vi "ParseData (SubVI).vi"(11 "read buffer":string) -> (3 "Array":bool[][](array[boolean]))   [LabVIEW 2021]
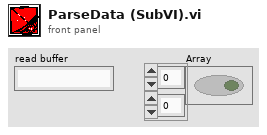
[diagram p1: front panel]
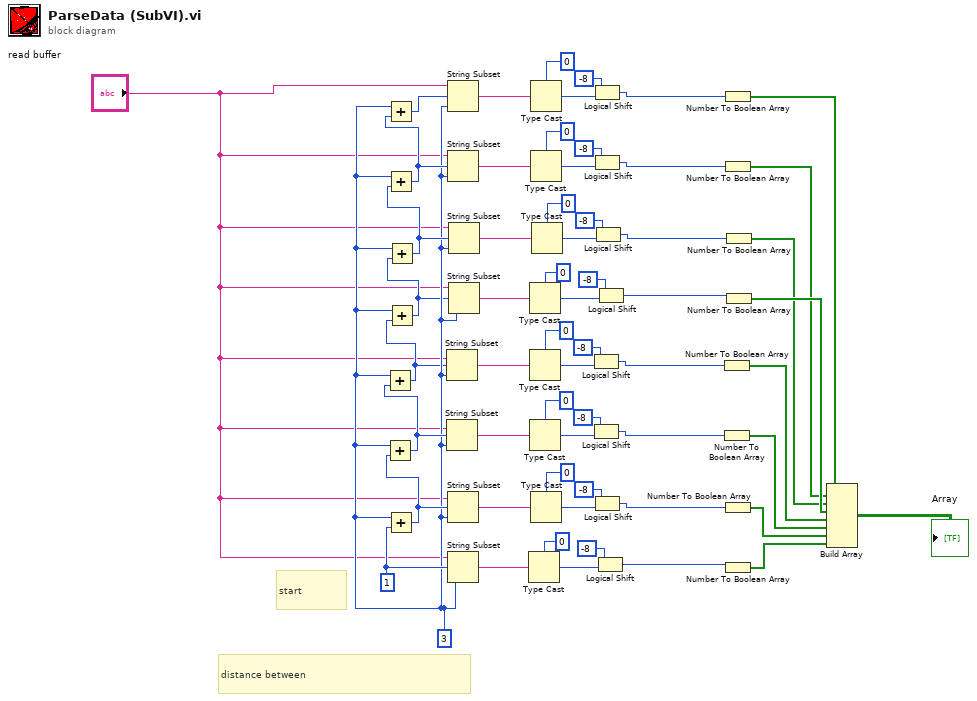
[diagram p0: block diagram]
diagram:
  w8 = 3 ("length (rest)")
  w46 = 1 ("offset (0)")
  # "start"
  # "distance between"
  n1 = Add(x=w8, y=w46) -> (x+y=w40:i32)
  n2 = Add(x=w8, y=w40) -> (x+y=w32:i32)
  n3 = Add(x=w8, y=w32) -> (x+y=w6:i32)
  n4 = Add(x=w8, y=w6) -> (x+y=w7:i32)
  n5 = Add(x=w8, y=w7) -> (x+y=w16:i32)
  n6 = Add(x=w8, y=w16) -> (x+y=w9:i32)
  n7 = Add(x=w8, y=w9) -> (x+y=w10:i32)
  n8 = String Subset(string="read buffer", offset (0)=w6, length (rest)=w8) -> (substring=w38:string)
  n9 = String Subset(string="read buffer", offset (0)=w32, length (rest)=w8) -> (substring=w45:string)
  n10 = String Subset(string="read buffer", offset (0)=w10, length (rest)=w8) -> (substring=w15:string)
  n11 = String Subset(string="read buffer", offset (0)=w9, length (rest)=w8) -> (substring=w21:string)
  n12 = String Subset(string="read buffer", offset (0)=w40, length (rest)=w8) -> (substring=w54:string)
  n13 = String Subset(string="read buffer", offset (0)=w46, length (rest)=w8) -> (substring=w56:string)
  n14 = String Subset(string="read buffer", offset (0)=w16, length (rest)=w8) -> (substring=w29:string)
  n15 = String Subset(string="read buffer", offset (0)=w7, length (rest)=w8) -> (substring=w31:string)
  n16 = Type Cast(type=u32 0, x=w56) -> (*(type *) &x=w48:u32)
  n17 = Type Cast(type=u32 0, x=w31) -> (*(type *) &x=w23:u32)
  n18 = Type Cast(type=u32 0 ("U16 Constant"), x=w38) -> (*(type *) &x=w35:u32)
  n19 = Type Cast(type=u32 0 ("U16 Constant"), x=w45) -> (*(type *) &x=w42:u32)
  n20 = Type Cast(type=u32 0 ("U16 Constant"), x=w15) -> (*(type *) &x=w12:u32)
  n21 = Type Cast(type=u32 0 ("U16 Constant"), x=w21) -> (*(type *) &x=w18:u32)
  n22 = Type Cast(type=u32 0 ("U16 Constant"), x=w54) -> (*(type *) &x=w51:u32)
  n23 = Type Cast(type=u32 0 ("U16 Constant"), x=w29) -> (*(type *) &x=w26:u32)
  n24 = Logical Shift(y=i16 -8, x=w35) -> (x << y=w34:u32)
  n25 = Logical Shift(y=i16 -8, x=w42) -> (x << y=w41:u32)
  n26 = Logical Shift(y=i16 -8, x=w12) -> (x << y=w11:u32)
  n27 = Logical Shift(y=i16 -8, x=w18) -> (x << y=w17:u32)
  n28 = Logical Shift(y=i16 -8, x=w51) -> (x << y=w50:u32)
  n29 = Logical Shift(y=i16 -8, x=w26) -> (x << y=w25:u32)
  n30 = Logical Shift(y=i16 -8, x=w48) -> (x << y=w47:u32)
  n31 = Logical Shift(y=i16 -8, x=w23) -> (x << y=w22:u32)
  n32 = Number To Boolean Array(number=w34) -> (Boolean array=w33:bool[])
  n33 = Number To Boolean Array(number=w41) -> (Boolean array=w39:bool[])
  n34 = Number To Boolean Array(number=w11) -> (Boolean array=w1:bool[])
  n35 = Number To Boolean Array(number=w17) -> (Boolean array=w2:bool[])
  n36 = Number To Boolean Array(number=w50) -> (Boolean array=w57:bool[])
  n37 = Number To Boolean Array(number=w47) -> (Boolean array=w58:bool[])
  n38 = Number To Boolean Array(number=w25) -> (Boolean array=w3:bool[])
  n39 = Number To Boolean Array(number=w22) -> (Boolean array=w4:bool[])
  n40 = Build Array(w1, w2, w3, w4, w33, w39, w57, w58) -> (→"Array":bool[][])
